vi "excel to graphe.vi"() -> ()   [LabVIEW 2021]
uses:
  <vilib>/Utility/file.llb/Read Delimited Spreadsheet (DBL).vi
panel:
  in  "file path (dialog if empty)":path
  out "XY Graph":cluster{"all rows":dbl[], "all rows":dbl[]}[](graph)
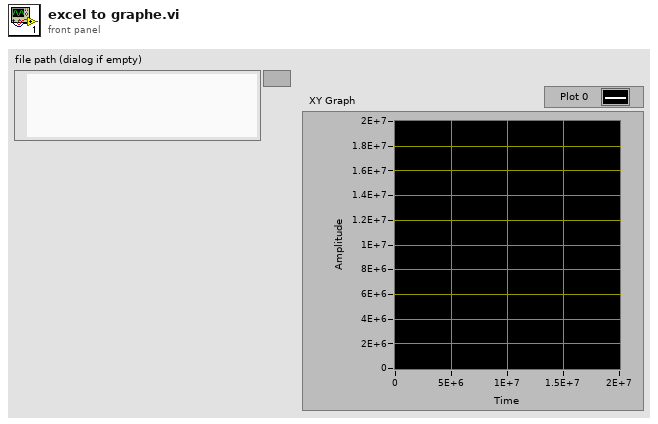
[diagram p1: front panel]
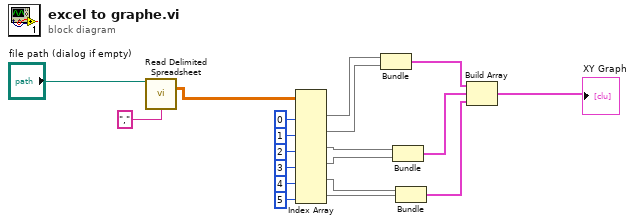
[diagram p0: block diagram]
diagram:
  n1 = call-poly <vilib>:"Read Delimited Spreadsheet.vi"("file path (dialog if empty)"="file path (dialog if empty)", "delimiter (\\t)"="," ("delimiter (\\t)")) -> ("all rows"=w17:dbl[][])  [unwired: 8 in, 5 out]
  n2 = Index Array(array=w17, index (col) #1=0 ("disabled index (col)"), index (col) #2=1 ("index (col)"), index (col) #3=2 ("index (col)"), index (col) #4=3 ("index (col)"), index (col) #5=4 ("index (col)"), index (col) #6=5 ("index (col)")) -> (element #1=w10:dbl[], element #2=w9:dbl[], element #3=w8:dbl[], element #4=w7:dbl[], element #5=w4:dbl[], element #6=w3:dbl[])  [unwired: 6 in]
  n3 = Bundle("all rows"=w10, "all rows"=w9) -> (w6:cluster{"all rows":dbl[], "all rows":dbl[]})  [unwired: 1 in]
  n4 = Bundle("all rows"=w8, "all rows"=w7) -> (w5:cluster{"all rows":dbl[], "all rows":dbl[]})  [unwired: 1 in]
  n5 = Bundle("all rows"=w4, "all rows"=w3) -> (w2:cluster{"all rows":dbl[], "all rows":dbl[]})  [unwired: 1 in]
  n6 = Build Array(w6, w5, w2) -> (→"XY Graph":cluster{"all rows":dbl[], "all rows":dbl[]}[])
